vi "Increment 2D Array Element.vi"(9 "index (col)":i32, 10 "index (row)":i32, 11 "array in":i32[][](array[numeric])) -> (3 "array out":i32[][](array[numeric]))   [LabVIEW 2019]
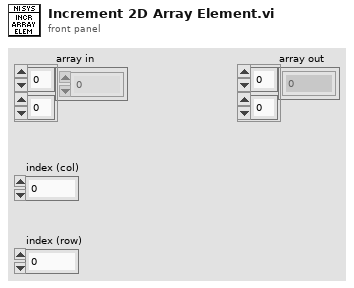
[diagram p1: front panel]
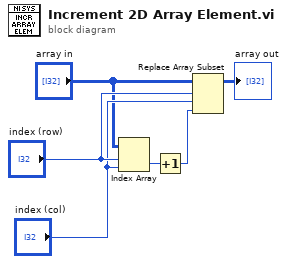
[diagram p0: block diagram]
diagram:
  n1 = Index Array(array="array in", index (row)="index (row)", index (col)="index (col)") -> (element=w3:i32)
  n2 = Increment(x=w3) -> (x+1=w4:i32)
  n3 = Replace Array Subset(array="array in", new element=w4, index (row)="index (row)", index (col)="index (col)") -> (→"array out":i32[][])
